vi "rudderAngle.vi"(4 "BoatHeading":dbl, 5 "YGoal":dbl, 6 "XGoal":dbl, 7 "Yboat":dbl, 8 "Xboat":dbl) -> (1 "Distance":dbl, 2 "Deflection":dbl, 3 "RudderAngle":dbl)   [LabVIEW 2012]
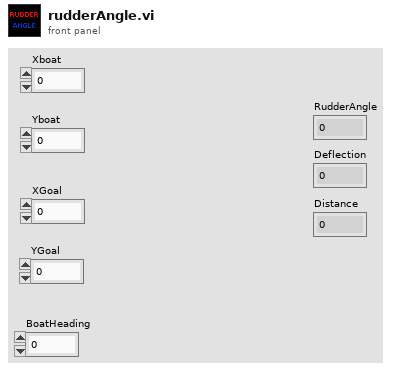
[diagram p1: front panel]
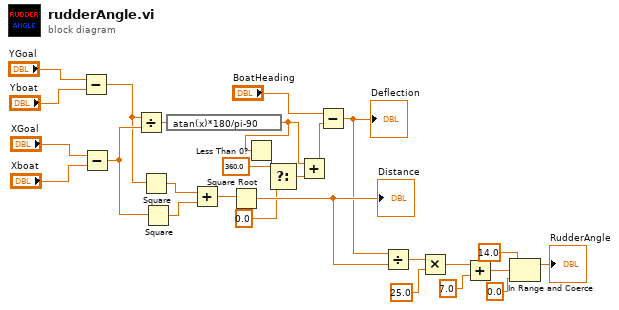
[diagram p0: block diagram]
diagram:
  n1 = Subtract(x="YGoal", y="Yboat") -> (x-y=w20:dbl)
  n2 = Subtract(x="XGoal", y="Xboat") -> (x-y=w21:dbl)
  n3 = Divide(x=w20, y=w21) -> (x/y=w23:dbl)
  n4 = Square(x=w20) -> (x^2=w18:dbl)
  n5 = Square(x=w21) -> (x^2=w19:dbl)
  n6 = expression code="atan(x)*180/pi-90"(w23) -> (w4:dbl)
  n7 = Add(x=w18, y=w19) -> (x+y=w17:dbl)
  n8 = Square Root(x=w17) -> (sqrt(x)=w16:dbl)
  "Distance" <- w16
  n9 = Less Than 0?(x=w4) -> (x < 0?=w6:bool)
  n10 = Select(t=360.0, s=w6, f=0.0) -> (s? t:f=w5:dbl)
  n11 = Add(x=w4, y=w5) -> (x+y=w3:dbl)
  n12 = Subtract(x="BoatHeading", y=w3) -> (x-y=w15:dbl)
  "Deflection" <- w15
  n13 = Divide(x=w15, y=w16) -> (x/y=w14:dbl)
  n14 = Multiply(x=w14, y=25.0) -> (x*y=w12:dbl)
  n15 = Add(x=w12, y=7.0) -> (x+y=w10:dbl)
  n16 = In Range and Coerce(upper limit=14.0, x=w10, lower limit=0.0) -> (coerced(x)=→"RudderAngle":dbl)  [unwired: 1 out]
